vi "Jacobi Iteration (rel residual).vi"(4 "max. iters":i32=10000, 5 "res. tol":dbl=1e-05, 6 "B":dbl[](array[numeric])=[6.0, 25.0, -11.0, 15.0], 7 "A":dbl[][](array[numeric])=[[10.0, -1.0, 2.0, 0.0], [-1.0, 11.0, -1.0, 3.0], [2.0, -1.0, 10.0, -1.0], [0.0, 3.0, -1.0, 8.0]]) -> (0 "Converged?":bool=TRUE, 1 "Iterations":i32=24, 3 "X":dbl[](array[numeric])=[1.0000000008366592, 1.9999999985888712, -0.9999999989100756, 0.9999999984529894])   [LabVIEW 2017]
panel:
  in  "Stop":bool
  out "Residual":sgl(graph)
  # "PN 21/10/17"
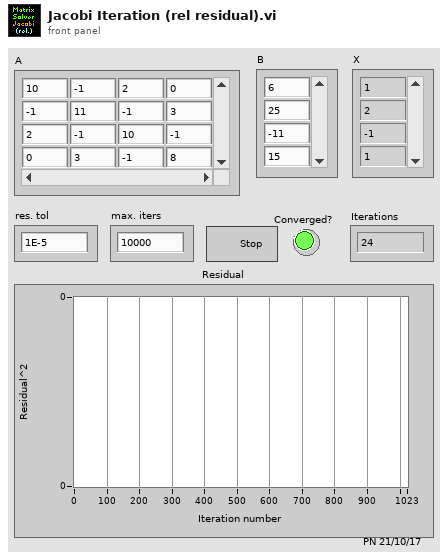
[diagram p1: front panel]
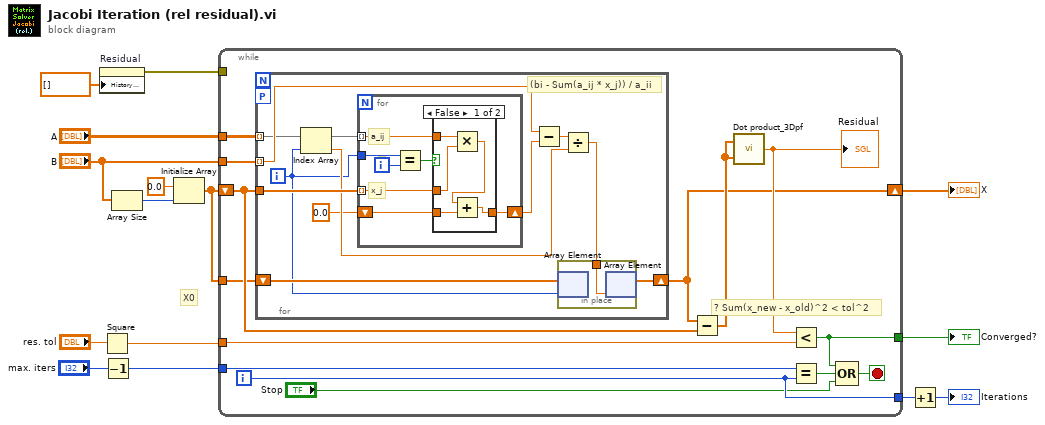
[diagram p0: block diagram]
diagram:
  # "X0"
  n1 = property on="Residual" class="WFChart (strict)"("History Data"=sgl[] []) -> (error out=w3:errorcluster)  [unwired: 2 in, 1 out]
  n2 = Square(x="res. tol") -> (x^2=w4:dbl)
  n3 = Decrement(x="max. iters") -> (x-1=w11:i32)
  n4 = Array Size(array="B") -> (size(s)=w14:i32)
  n5 = Initialize Array(0.0 ("element"), w14) -> (w2:dbl[])
  n6 = while {
    tunnel: "A" -> [w29]
    tunnel: "B" -> [w28]
    tunnel: w4 -> [w26]
    shift-right: [w19] -> w7
    shift-left: w2 -> [w27]
    tunnel: w11 -> [w24]
    tunnel: [w23] -> w10
    tunnel: [w17] -> w1
    tunnel: w3 -> [_]
    tunnel: w2 -> [w20]
    i -> [w23]
    stop <- w25 stop-if-true
    # "? Sum(x_new - x_old)^2 < tol^2"
    n7 = for {
      tunnel: w28 -> [w39] mode=indexing
      tunnel: w29 -> [w36] mode=indexing
      tunnel: w27 -> [w40]
      workers-P: _ -> [_]
      shift-right: [w32] -> w19
      shift-left: w20 -> [w33]
      i -> [w31]
      # "(bi - Sum(a_ij * x_j)) / a_ii"
      n8 = Index Array(array=w36, index=w31) -> (element=w37:dbl)
      n9 = for {
        tunnel: w31 -> [w47]
        tunnel: w36 -> [w45] mode=indexing
        tunnel: w40 -> [w44] mode=indexing
        shift-right: [w42] -> w34
        shift-left: 0.0 ("element") -> [w43]
        i -> [w48]
        # "x_j"
        # "a_ij"
        # "j"
        n10 = Equal?(x=w47, y=w48) -> (x = y?=w46:bool)
        n11 = case shown="False" w46 {
          tunnel: w45 -> [w53 _]
          tunnel: w44 -> [w52 _]
          tunnel: w43 -> [w51 w54]
          tunnel: [w50 w54] -> w42
          frame False {
            n12 = Multiply(x=w53, y=w52) -> (x*y=w49:dbl)
            n13 = Add(x=w49, y=w51) -> (x+y=w50:dbl)
          }
          frame True {
          }
        }
      }
      n14 = Subtract(x=w39, y=w34) -> (x-y=w38:dbl)
      n15 = Divide(x=w38, y=w37) -> (x/y=w30:dbl)
      n16 = in-place {
        in-place-border: w30 -> [w41]
        n17 = in-place-array #1(w33, w31) -> ()  [unwired: 1 out]
        n18 = in-place-array #1(w41) -> (w32:dbl[])  [unwired: 1 out]
      }
    }
    n19 = Subtract(x=w19, y=w27) -> (x-y=w22:dbl[])
    n20 = call "Dot product_3Dpf.vi"("B"=w22, "A"=w22) -> ("A . B"=w21:sgl)
    "Residual" <- w21
    n21 = Less?(x=w21, y=w26) -> (x < y?=w17:bool)
    n22 = Equal?(x=w24, y=w23) -> (x = y?=w18:bool)
    n23 = Compound Arithmetic op=OR(w17, w18, "Stop") -> (w25:bool)
  }
  "X" <- w7
  "Converged?" <- w1
  n24 = Increment(x=w10) -> (x+1=→"Iterations":i32)
